vi "Write Tx Values and Read Rx Values Until Equal.vi"(4 "tolerance (0.01)":dbl=0.01, 6 "Tx values":dbl[](array[numeric]), 7 "timeout (1000 ms)":i32=1000, 8 "error in":errorcluster, 9 "Rx aliases":string[](array[string]), 10 "Tx aliases":string[](array[string]), 11 "workspace manager in":T1) -> (0 "error out":errorcluster, 2 "values equal":bool, 3 "workspace manager out":T1)   [LabVIEW 2027, in "VeriStandTestUtilities.lvlib"]
uses:
  VeriStandTestUtilities.lvlib
  <vilib>/NI VeriStand/Execution/Workspace/WorkspaceAPI.ctl
  C:/NetCoreDLL/NationalInstruments.VeriStand.ClientAPI.dll
  NetCoreDLL/NationalInstruments.VeriStand.ClientAPI.dll
  <vilib>/NI VeriStand/Execution/Workspace/NI VeriStand - Set Multiple Channel Values.vi
  <vilib>/NI VeriStand/Execution/Workspace/NI_VS Workspace ExecutionAPI.lvlib
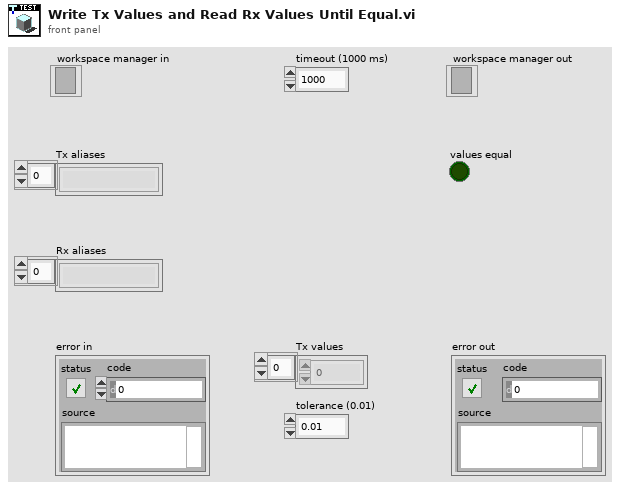
[diagram p1: front panel]
types:
  T1 = typedef "NI_VS Workspace ExecutionAPI.lvlib/WorkspaceAPI.ctl" = refnum<k39>
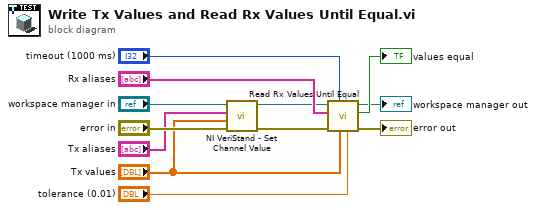
[diagram p0: block diagram]
diagram:
  n1 = call-poly <vilib>:"NI VeriStand - Set Channel Value.vi"("error in (no error)"="error in", "Values"="Tx values", "Channels"="Tx aliases", "WorkspaceManager in"="workspace manager in") -> ("error out"=w6:errorcluster, "WorkspaceManager out"=w7:T1)  [unwired: 6 in]
  n2 = call "Read Rx Values Until Equal.vi"("tolerance (0.01)"="tolerance (0.01)", "expected values"="Tx values", "timeout (1000 ms)"="timeout (1000 ms)", "error in"=w6, "Rx aliases"="Rx aliases", "workspace manager in"=w7) -> ("error out"=→"error out":errorcluster, "values equal expected"=→"values equal":bool, "workspace manager out"=→"workspace manager out":T1)  [unwired: 3 in]
